vi "DAQ设置.vi"(0 "引用句柄输入":refnum<k21>, 1 "physical channels":tag[](array[tag]) caption="物理通道", 5 "error out":errorcluster caption="错误输出") -> (14 "task out":refnum<k21>, 19 "error IO":errorcluster)   [LabVIEW 2018]
uses:
  <vilib>/DAQmx/create/channels.llb/DAQmx Create Channel (AI-Sound Pressure-Microphone).vi
  <vilib>/DAQmx/configure/timing.llb/DAQmx Timing (Sample Clock).vi
  <resource>/objmgr/daqmx.rc
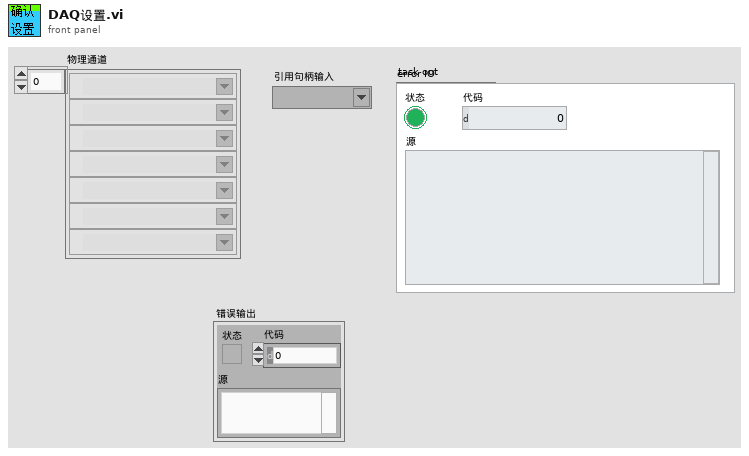
[diagram p1: front panel]
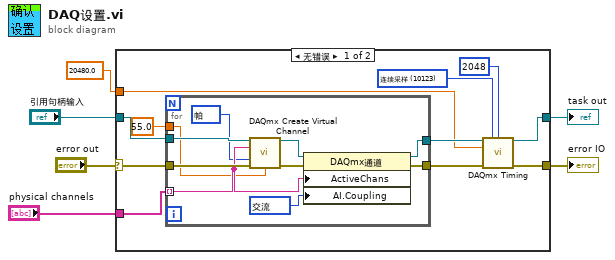
[diagram p0: block diagram]
diagram:
  n1 = case shown="无错误" "error out" {
    selector: "error out" -> [w16 w29]
    tunnel: "引用句柄输入" -> [w17 w28]
    tunnel: [w11 w28] -> w5
    tunnel: [w10 w29] -> w3
    tunnel: 20480.0 ("rate") -> [w9 _]
    tunnel: "physical channels" -> [w8 _]
    frame No Error {
      w13 = 10123 items=["有限采样"=10178, "连续采样"=10123, "硬件定时单点"=12522] ("sample mode")
      n2 = for {
        tunnel: w17 -> [w27]
        tunnel: 55.0 -> [w18]
        tunnel: [w24] -> w15
        tunnel: [w22] -> w14
        tunnel: w16 -> [w26]
        tunnel: w8 -> [w20] mode=indexing
        w19 = 10081 items=["帕"=10081, "来自自定义换算"=10065] ("units")
        w21 = 10045 items=["交流"=10045, "直流"=10050, "GND"=10066] ("AI.Coupling")
        n3 = call-poly <vilib>:"DAQmx Create Virtual Channel.vi"("task in"=w27, "physical channels"=w20, "units"=w19, "error in"=w26, "microphone sensitivity"=w18) -> ("task out"=w25:refnum<k21>, "error out"=w23:errorcluster)  [unwired: 9 in]
        n4 = property class="DAQmx通道"(reference=w25, error in=w23, "ActiveChans"=w20, "AI.Coupling"=w21) -> (reference out=w24:refnum<k21>, error out=w22:errorcluster)
      }
      n5 = call-poly <vilib>:"DAQmx Timing.vi"("task/channels in"=w15, "sample mode"=w13, "samples per channel"=2048, "rate"=w9, "error in"=w14) -> ("task out"=w11:refnum<k21>, "error out"=w10:errorcluster)  [unwired: 9 in]
    }
    frame Error {
    }
  }
  "task out" <- w5
  "error IO" <- w3
